vi "Update Event List.vi"(8 "error in (no error)":errorcluster, 11 "UI Controller in":refnum<class "UI Controller.lvclass">) -> (0 "error out":errorcluster, 3 "UI Controller out":refnum<class "UI Controller.lvclass">)   [LabVIEW 2019, in "UI Controller.lvlib" / "UI Controller.lvclass"]
uses:
  UI Controller.lvclass
  <vilib>/Utility/sysdir.llb/System Directory Type.ctl
  UI Controller.lvclass/UI Controller.ctl
  <vilib>/GPower/Files & Folders/Library/GPFilesFolders.lvlib
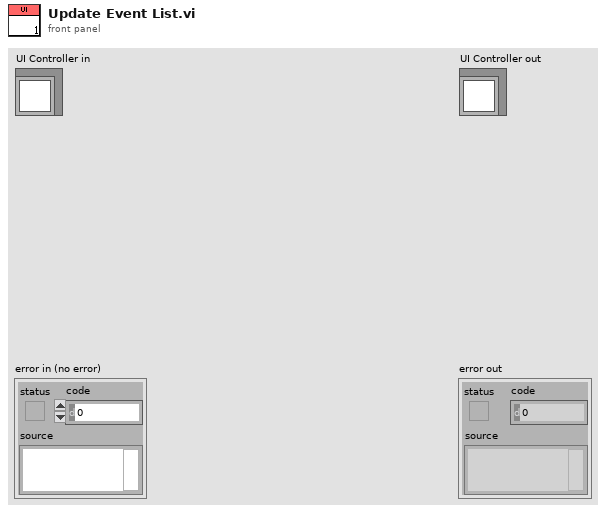
[diagram p1: front panel]
types:
  T1 = typedef "System Directory Type.ctl" = i32
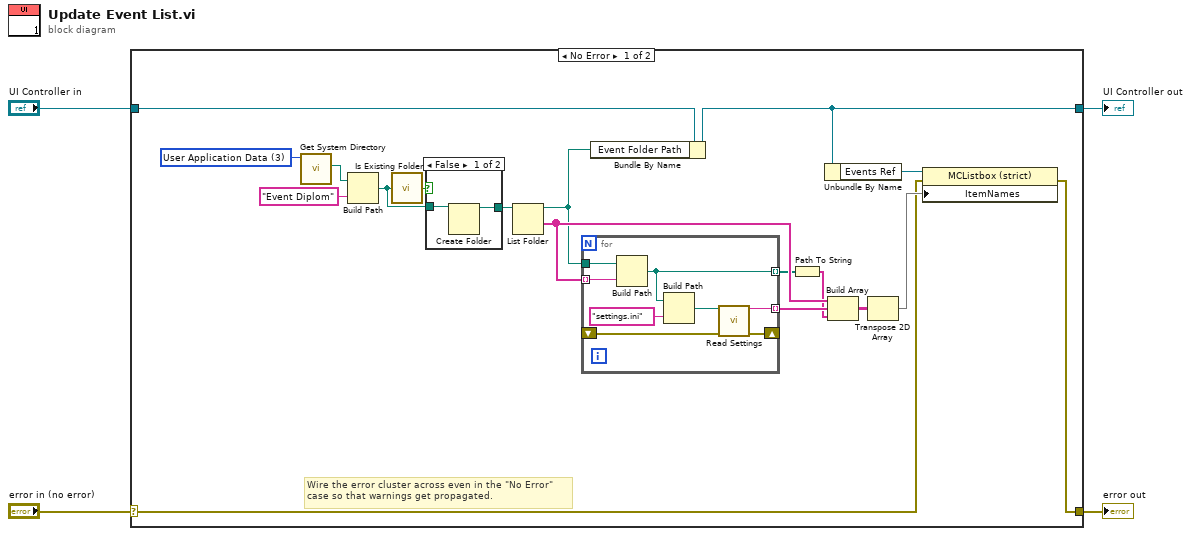
[diagram p0: block diagram]
diagram:
  n1 = case shown="No Error" "error in (no error)" {
    selector: "error in (no error)" -> [w9 w35]
    tunnel: [w8 w35] -> w3
    tunnel: [w7 w34] -> w1
    tunnel: "UI Controller in" -> [w6 w34]
    frame No Error {
      w22 = T1 3 items=["User Home"=0, "User Desktop"=1, "User Documents"=2, "User Application Data"=3, "User Preferences"=4, "User Temporary"=5, "Public Documents"=6, "Public Application Data"=7, "Public Preferences"=8, "Public Cache"=13, "System Core Libraries"=9, "System Installed Libraries"=10, "Application Files"=11, "Boot Volume Root"=12] ("system directory type")
      # "Wire the error cluster across even in the \"No Error\"\ncase so that warnings get propagated."
      n2 = call <vilib>:"Get System Directory.vi"("system directory type"=w22) -> ("system directory"=w21:path)  [unwired: 10 in]
      n3 = Build Path(base path=w21, name or relative path="Event Diplom") -> (appended path=w19:path)
      n4 = call <vilib>:"Is Existing Folder.vi"("Folder Path"=w19) -> ("Existing Folder?"=w18:bool)  [unwired: 4 in]
      n5 = case shown="False" w18 {
        tunnel: w19 -> [w32 w33]
        tunnel: [w31 w33] -> w17
        frame False {
          n6 = Create Folder(path (use dialog)=w32) -> (created path=w31:path)  [unwired: 2 in, 2 out]
        }
        frame True {
        }
      }
      n7 = List Folder(path=w17) -> (path out=w5:path, folder names=w16:string[])  [unwired: 3 in, 2 out]
      n8 = for {
        tunnel: w16 -> [w29] mode=indexing
        tunnel: w5 -> [w30]
        tunnel: [w26] -> w15 mode=indexing
        shift-right: [w25] -> _
        shift-left: _ -> [w24]
        tunnel: [w23] -> w13 mode=indexing
        n9 = Build Path(base path=w30, name or relative path=w29) -> (appended path=w23:path)
        n10 = Build Path(base path=w23, name or relative path="settings.ini") -> (appended path=w27:path)
        n11 = call "Read Settings.vi"("Path"=w27, "Error in"=w24) -> ("Description"=w26:string, "Error out"=w25:errorcluster)  [unwired: 12 in]
      }
      n12 = Bundle By Name(cluster=w6, "Event Folder Path"=w5) -> (w7:refnum<class "UI Controller.lvclass">)
      n13 = Path To String(path=w13) -> (string=w12:string[])
      n14 = Unbundle By Name(w7) -> ("Events Ref"=w11:refnum<vi>)
      n15 = Build Array(w16, w15, w12) -> (w14:string[][])
      n16 = Transpose 2D Array(2D array=w14) -> (transposed array=w10:string[][])
      n17 = property class="MCListbox (strict)"(reference=w11, error in=w9, "ItemNames"=w10) -> (error out=w8:errorcluster)  [unwired: 1 out]
    }
    frame Error {
    }
  }
  "error out" <- w3
  "UI Controller out" <- w1
